vi "getSoundPath.vi"(8 "error in (no error)":errorcluster, 11 "SoundDeviceData in":refnum<class "SoundDeviceData.lvclass">) -> (0 "error out":errorcluster, 2 "Path":path, 3 "SoundDeviceData out":refnum<class "SoundDeviceData.lvclass">)   [LabVIEW 2011, in "DataMappers.lvlib" / "SoundDeviceData.lvclass"]
uses:
  SoundDeviceData.lvclass
  Filing/FileNeologist/FileNeologist.lvclass
  Filing.lvlib
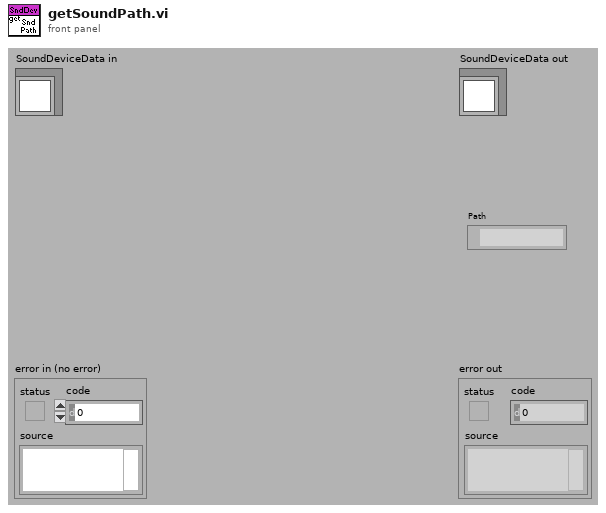
[diagram p1: front panel]
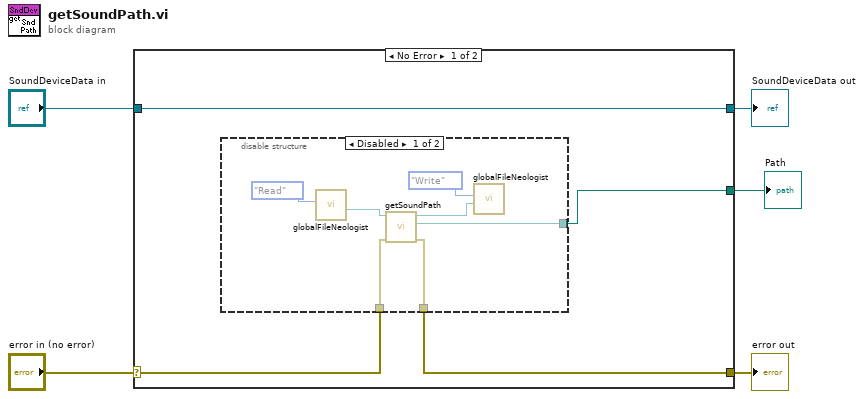
[diagram p0: block diagram]
diagram:
  n1 = case shown="No Error" "error in (no error)" {
    selector: "error in (no error)" -> [w7 w19]
    tunnel: [w6 w19] -> w4
    tunnel: [w9 w18] -> w2
    tunnel: "SoundDeviceData in" -> [w9 w18]
    tunnel: [w8 _] -> w1
    frame No Error {
      n2 = disable-structure shown="Disabled" {
        disable-tunnel: [w12 _] -> w8
        disable-tunnel: w7 -> [w11 w17]
        disable-tunnel: [w10 w17] -> w6
        frame Disabled {
          n3 = call "globalFileNeologist.vi"("Action"=enum16{"Write", "Read"}."Read") -> ("FileNeologist out"=w16:refnum<class "FileNeologist.lvclass">)  [unwired: 10 in]
          n4 = call "getSoundPath.vi"("error in (no error)"=w11, "FileNeologist in"=w16) -> ("error out"=w10:errorcluster, "Path"=w12:path, "FileNeologist out"=w13:refnum<class "FileNeologist.lvclass">)  [unwired: 7 in]
          n5 = call "globalFileNeologist.vi"("FileNeologist in"=w13, "Action"=enum16{"Write", "Read"}."Write") -> ()  [unwired: 9 in, 1 out]
        }
        frame Enabled {
        }
      }
    }
    frame Error {
    }
  }
  "error out" <- w4
  "SoundDeviceData out" <- w2
  "Path" <- w1
